vi "AtSpectrograph_issueCommand_changeDisperser.vi"(8 "error in (no error)":errorcluster, 11 "command_changeDisperser_Ctl":T1) -> (0 "error out":errorcluster, 2 "function return":i32, 3 "command_changeDisperser_Ctl out":T1)   [LabVIEW 2016, in "SALLV_AtSpectrograph.lvlib"]
doc: "int AtSpectrograph_shm_issueCommand_changeDisperserLV(AtSpectrograph_command_changeDisperserLV *command_changeDisperser_Ctl );"
uses:
  SALLV_AtSpectrograph.lvlib
  DataTypes/command_changeDisperser.ctl
  SALLV_AtSpectrograph.so
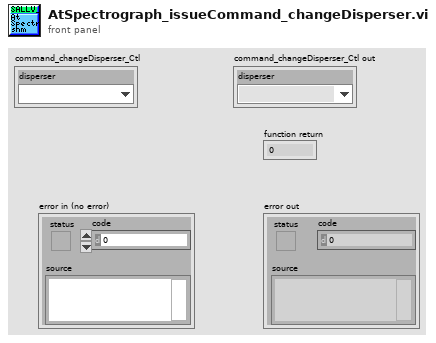
[diagram p1: front panel]
types:
  T1 = typedef "SALLV_AtSpectrograph.lvlib/command_changeDisperser.ctl" = cluster{"disperser":enum32{"", "Slot0", "Slot1", "Slot2", "Slot3"}}
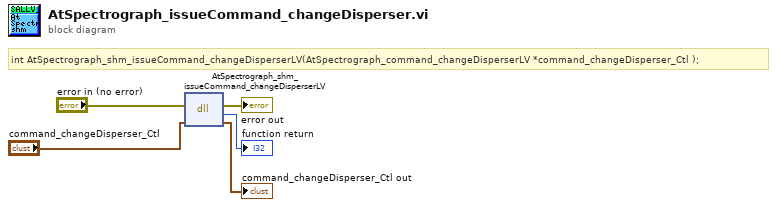
[diagram p0: block diagram]
diagram:
  # "int AtSpectrograph_shm_issueCommand_changeDisperserLV(AtSpectrograph_command_changeDisperserLV *command_changeDisperser_Ctl );"
  n1 = dll-call lib="home/harini/tcs/temp/SALLV_AtSpectrograph/SALLV_AtSpectrograph.*" fn="AtSpectrograph_shm_issueCommand_changeDisperserLV"(error in="error in (no error)", "command_changeDisperser_Ctl"="command_changeDisperser_Ctl") -> (error out=→"error out":errorcluster, →"function return":i32, "command_changeDisperser_Ctl"=→"command_changeDisperser_Ctl out":T1)  [unwired: 2 in, 1 out]
